vi "HH_AccumCounts.vi"(0 "Data In":u32[](array[numeric]), 1 "Reset":bool, 5 "Data Count":i32, 11 "Acc X Overflows":i32=25) -> (4 "Histograms":i32[][](array[numeric]), 8 "Accum Counts":u32[](array[numeric]), 10 "Acc Time Ok":bool, 13 "Total Oveflow Count":u64, 14 "Num Records Total":i32)   [LabVIEW 2011]
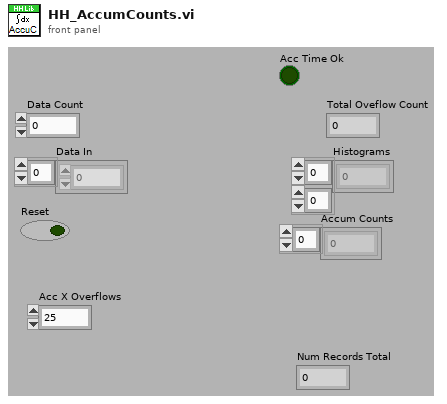
[diagram p1: front panel]
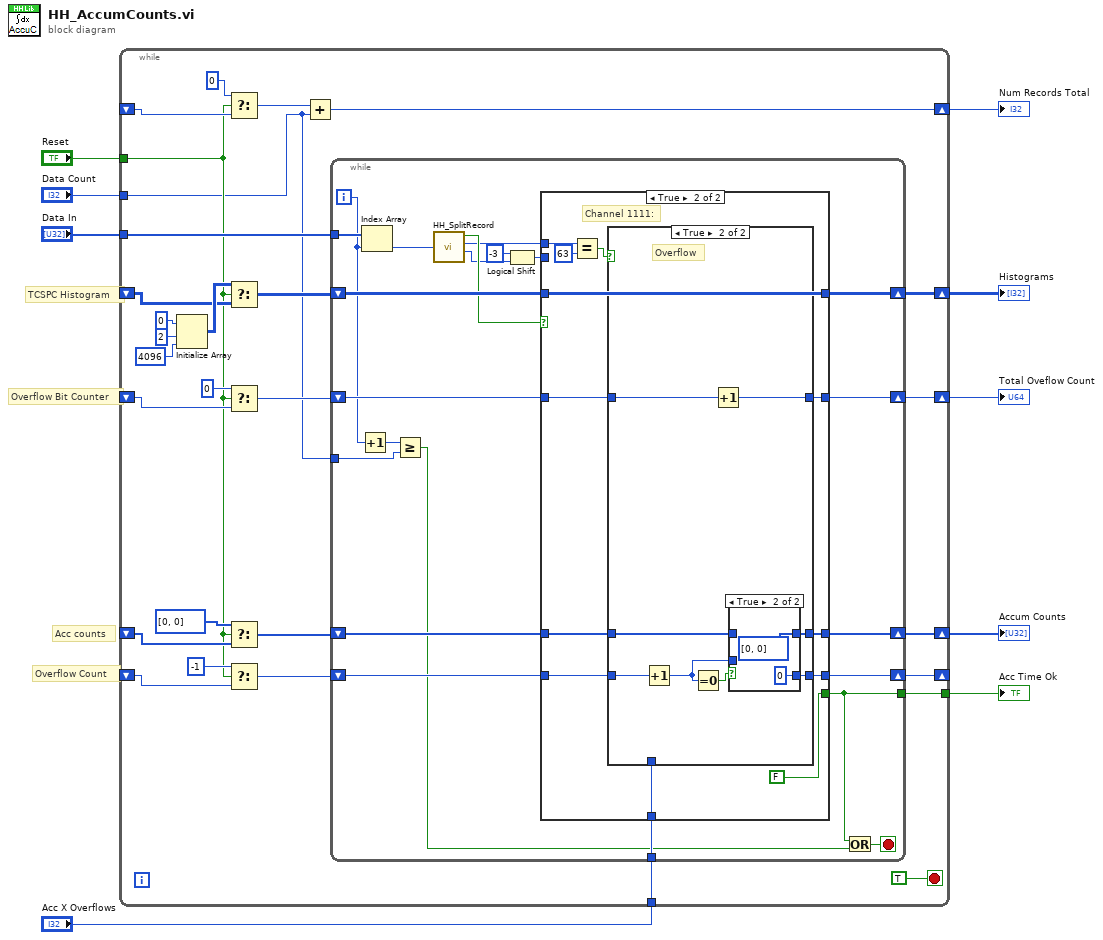
[diagram p0: block diagram]
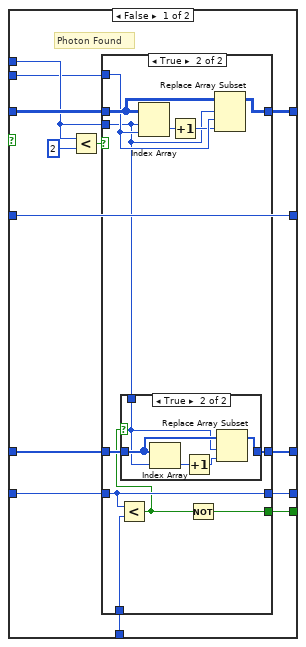
[diagram p2: hidden frame]
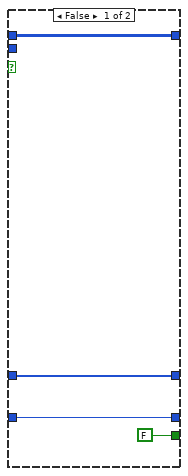
[diagram p3: hidden frame]
diagram:
  # "Overflow Count"
  # "Acc counts"
  # "TCSPC Histogram"
  # "Overflow Bit Counter"
  n1 = while {
    tunnel: "Data In" -> [w36]
    shift-right: [w37] -> w9
    shift-left: _ -> [w32]
    tunnel: "Reset" -> [w12]
    shift-right: [w29] -> w3
    shift-left: _ -> [w28]
    shift-right: [w26] -> w2
    shift-left: _ -> [w25]
    shift-right: [w23] -> _
    shift-left: _ -> [w22]
    tunnel: "Acc X Overflows" -> [w21]
    tunnel: "Data Count" -> [w11]
    shift-right: [w17] -> w4
    shift-left: _ -> [w19]
    tunnel: [w10] -> w1
    stop <- TRUE stop-if-true
    n2 = Initialize Array(0 ("element"), 2 ("dimension size"), 4096 ("dimension size")) -> (w33:i32[][])
    n3 = Select(t=0 ("Data Count 2"), s=w12, f=w19) -> (s? t:f=w18:i32)
    n4 = Select(t=w33, s=w12, f=w32) -> (s? t:f=w34:i32[][])
    n5 = Select(t=u64 0, s=w12, f=w28) -> (s? t:f=w30:u64)
    n6 = Select(t=u32[] [0, 0] ("initialized array"), s=w12, f=w25) -> (s? t:f=w27:u32[])
    n7 = Select(t=-1, s=w12, f=w22) -> (s? t:f=w24:i32)
    n8 = Add(x=w18, y=w11) -> (x+y=w17:i32)
    n9 = while {
      tunnel: w36 -> [w52]
      shift-right: [w59] -> w37
      shift-left: w34 -> [w60]
      shift-right: [w57] -> w29
      shift-left: w30 -> [w58]
      shift-right: [w55] -> w26
      shift-left: w27 -> [w56]
      shift-right: [w53] -> w23
      shift-left: w24 -> [w54]
      tunnel: w21 -> [w51]
      tunnel: w11 -> [w48]
      tunnel: [w45] -> w10
      i -> [w50]
      stop <- w46 stop-if-true
      n10 = Increment(x=w50) -> (x+1=w49:i32)
      n11 = Index Array(array=w52, index=w50) -> (element=w44:u32)
      n12 = Greater Or Equal?(x=w49, y=w48) -> (x >= y?=w47:bool)
      n13 = call "HH_SplitRecord.vi"("Record in"=w44) -> ("Special"=w43:bool, "channel"=w39:i32, "time"=w41:i32)  [unwired: 1 out]
      n14 = Logical Shift(y=i8 -3, x=w41) -> (x << y=w40:i32)
      n15 = case shown="True" w43 {
        tunnel: w60 -> [w73 w105]
        tunnel: w39 -> [w62 w97]
        tunnel: [w72 w105] -> w59
        tunnel: w40 -> [w61 _]
        tunnel: w58 -> [w71 w107]
        tunnel: [w71 w106] -> w57
        tunnel: w56 -> [w70 w103]
        tunnel: [w69 w101] -> w55
        tunnel: w54 -> [w65 w104]
        tunnel: [w64 w102] -> w53
        tunnel: w51 -> [w66 w100]
        tunnel: [w63 FALSE] -> w45
        frame False {
          # "Photon Found"
          n16 = Less?(x=w62, y=2) -> (x < y?=w68:bool)
          n17 = case shown="True" w68 {
            tunnel: w73 -> [w77 w89]
            tunnel: [w77 w88] -> w72
            tunnel: w61 -> [_ w87]
            tunnel: w62 -> [_ w82]
            tunnel: w70 -> [w76 w86]
            tunnel: [w76 w85] -> w69
            tunnel: w66 -> [_ w81]
            tunnel: w65 -> [w75 w80]
            tunnel: [w75 w80] -> w64
            tunnel: [FALSE w78] -> w63
            frame False {
            }
            frame True {
              n18 = Less?(x=w80, y=w81) -> (x < y?=w79:bool)
              n19 = case shown="True" w79 {
                tunnel: w86 -> [w90 w95]
                tunnel: [w90 w94] -> w85
                tunnel: w82 -> [_ w91]
                frame False {
                }
                frame True {
                  n20 = Index Array(array=w95, index=w91) -> (element=w93:u32)
                  n21 = Increment(x=w93) -> (x+1=w92:u32)
                  n22 = Replace Array Subset(array=w95, new element=w92, index=w91) -> (w94:u32[])
                }
              }
              n23 = Index Array(array=w89, index (row)=w82, index (col)=w87) -> (element=w84:i32)
              n24 = Increment(x=w84) -> (x+1=w83:i32)
              n25 = Not(x=w79) -> (.not. x?=w78:bool)
              n26 = Replace Array Subset(array=w89, new element=w83, index (row)=w82, index (col)=w87) -> (w88:i32[][])
            }
          }
        }
        frame True {
          # "Channel 1111:"
          n27 = Equal?(x=w97, y=63) -> (x = y?=w96:bool)
          n28 = case shown="True" w96 {
            tunnel: w107 -> [w110 w118]
            tunnel: [w110 w117] -> w106
            tunnel: w104 -> [w109 w112]
            tunnel: w103 -> [w108 w114]
            tunnel: [w109 w115] -> w102
            tunnel: [w108 w113] -> w101
            tunnel: w100 -> [_ _]
            frame False {
              # "Trigger Signal"
            }
            frame True {
              # "Overflow"
              n29 = Increment(x=w112) -> (x+1=w111:i32)
              n30 = Equal To 0?(x=w111) -> (x = 0?=w116:bool)
              n31 = Increment(x=w118) -> (x+1=w117:u64)
              n32 = case shown="True" w116 {
                tunnel: w111 -> [w120 _]
                tunnel: [w120 0] -> w115
                tunnel: w114 -> [w119 _]
                tunnel: [w119 u32[] [0, 0] ("initialized array")] -> w113
                frame False {
                }
                frame True {
                }
              }
            }
          }
        }
      }
      n33 = Or(x=w45, y=w47) -> (x .or. y?=w46:bool)
    }
  }
  "Histograms" <- w9
  "Num Records Total" <- w4
  "Total Oveflow Count" <- w3
  "Accum Counts" <- w2
  "Acc Time Ok" <- w1
